vi "Pump Status Pump Module.vi"(8 "error in (no error)":errorcluster, 11 "?":T1={"State"=enum."Idle", "Start Time"=timestamp(0 s since 1904-01-01), "Configuration"={"Cycle Period"=0.0, "Ismatech"={"VISA resource name"="", "Simulated?"=FALSE, "Pump Number"=1.0, "Reverse?"=FALSE}, "Masterflex"={"VISA resource name"="", "Simulated?"=FALSE, "Pump Number"=1.0, "Reverse?"=FALSE}, "Manual Entry"=0.0, "VICI Settings"={"VISA resource name"="", "Simulated?"=FALSE, "Pump Letter"="", "Reverse?"=FALSE}, "Output Device"=enum."VICI", "Tacmina Settings"={"Analog DAQ Task"="", "Digital DAQ Task"=""}, "KNF SIMDOS Settings"={"VISA resource name"="", "Simulated?"=TRUE}, "ASIA Pump C"={"ASIA Pump #"=0, "channel"=0, "Simulated"=FALSE}, "FLOM Settings"={"VISA resource name"="", "Simulated?"=TRUE, "Pump Number"=0.0}, "Pump Calibration File"=path "", "Calibration Slope"=0.0, "Calibration Y Intercept"=0.0, "Pump Cal Enum"=0, "SSI PR Settings"={"VISA resource name"="", "Simulated?"=FALSE}}, "Current Time"=timestamp(0 s since 1904-01-01), "First Iteration"=FALSE, "Data"={"Pump Speed"=0.0, "Pump Pressure"=0.0, "Pump Flow"=0.0}, "Process Name"="", "Pump On?"=enum."Off", "Output Error"=FALSE, "Log Started"=FALSE, "Overpressure Alarming"=FALSE} {"Configuration"."ASIA Pump C"."channel" min=0 max=1 step=1; "Configuration"."Masterflex"."Pump Number" min=1.0 max=20.0 step=1.0; "Configuration"."Ismatech"."Pump Number" min=1.0 max=20.0 step=1.0}) -> (0 "error out":errorcluster, 3 "State out":T1={"State"=enum."Idle", "Start Time"=timestamp(0 s since 1904-01-01), "Configuration"={"Cycle Period"=0.0, "Ismatech"={"VISA resource name"="", "Simulated?"=FALSE, "Pump Number"=1.0, "Reverse?"=FALSE}, "Masterflex"={"VISA resource name"="", "Simulated?"=FALSE, "Pump Number"=1.0, "Reverse?"=FALSE}, "Manual Entry"=0.0, "VICI Settings"={"VISA resource name"="", "Simulated?"=FALSE, "Pump Letter"="", "Reverse?"=FALSE}, "Output Device"=enum."Ismatec ISM 831C", "Tacmina Settings"={"Analog DAQ Task"="", "Digital DAQ Task"=""}, "KNF SIMDOS Settings"={"VISA resource name"="", "Simulated?"=TRUE}, "ASIA Pump C"={"ASIA Pump #"=0, "channel"=0, "Simulated"=FALSE}, "FLOM Settings"={"VISA resource name"="", "Simulated?"=TRUE, "Pump Number"=0.0}, "Pump Calibration File"=path "", "Calibration Slope"=0.0, "Calibration Y Intercept"=0.0, "Pump Cal Enum"=0, "SSI PR Settings"={"VISA resource name"="", "Simulated?"=FALSE}}, "Current Time"=timestamp(0 s since 1904-01-01), "First Iteration"=FALSE, "Data"={"Pump Speed"=0.0, "Pump Pressure"=0.0, "Pump Flow"=0.0}, "Process Name"="", "Pump On?"=enum."Off", "Output Error"=FALSE, "Log Started"=FALSE, "Overpressure Alarming"=FALSE} {"Configuration"."ASIA Pump C"."channel" min=0 max=1 step=1; "Configuration"."Masterflex"."Pump Number" min=1.0 max=20.0 step=1.0; "Configuration"."Ismatech"."Pump Number" min=1.0 max=20.0 step=1.0})   [LabVIEW 2018, in "Pump Module.lvlib"]
uses:
  Pump Module.lvlib
  Measure Instrument/State Cluster.ctl
  Measure Instrument/State Enum.ctl
  Pump Module Settings Cluster.ctl
  Ismatec ISM 831C/Controls/Ismatech Settings Cluster.ctl
  Masterflex 7550-30/Controls/Settings Cluster.ctl
  VICI M50 Party Mode/Settings Cluster.ctl
  Measure Instrument/PID 2 Output Enum.ctl
  Tacmina QI/Tacmina QI DAQ Setting.ctl
  KNF Pump/Settings Cluster plus SIMDOS.ctl
  ASIA Pump/Pump Settings.ctl
  FLOM Pump/Settings Cluster.ctl
  SSI PR Class/SSI PR Settings Cluster.ctl
  Tag VIs/Tag FGV Operation Enum.ctl
  Ismatec ISM 831C/Ismatec ISM 831C.lvlib
  Masterflex 7550-30/Masterflex 7550-30.lvlib
  Shared Variables/Dynamic Shared Variables.lvlib
  Measure Instrument/Pump Module Engine.lvlib
  Tacmina QI/Tacmina QI.lvlib
  KNF Pump/KNF SIMDOS.lvlib
  VICI M50 Party Mode/VICI M6 M50 Party Mode.lvlib
  FLOM Pump/FLOM Pump.lvlib
  ASIA Pump.lvlib
  SSI PR Class/SSI PR Pump.lvlib
panel:
  # "Output Instruments"
  # "Output Instruments"
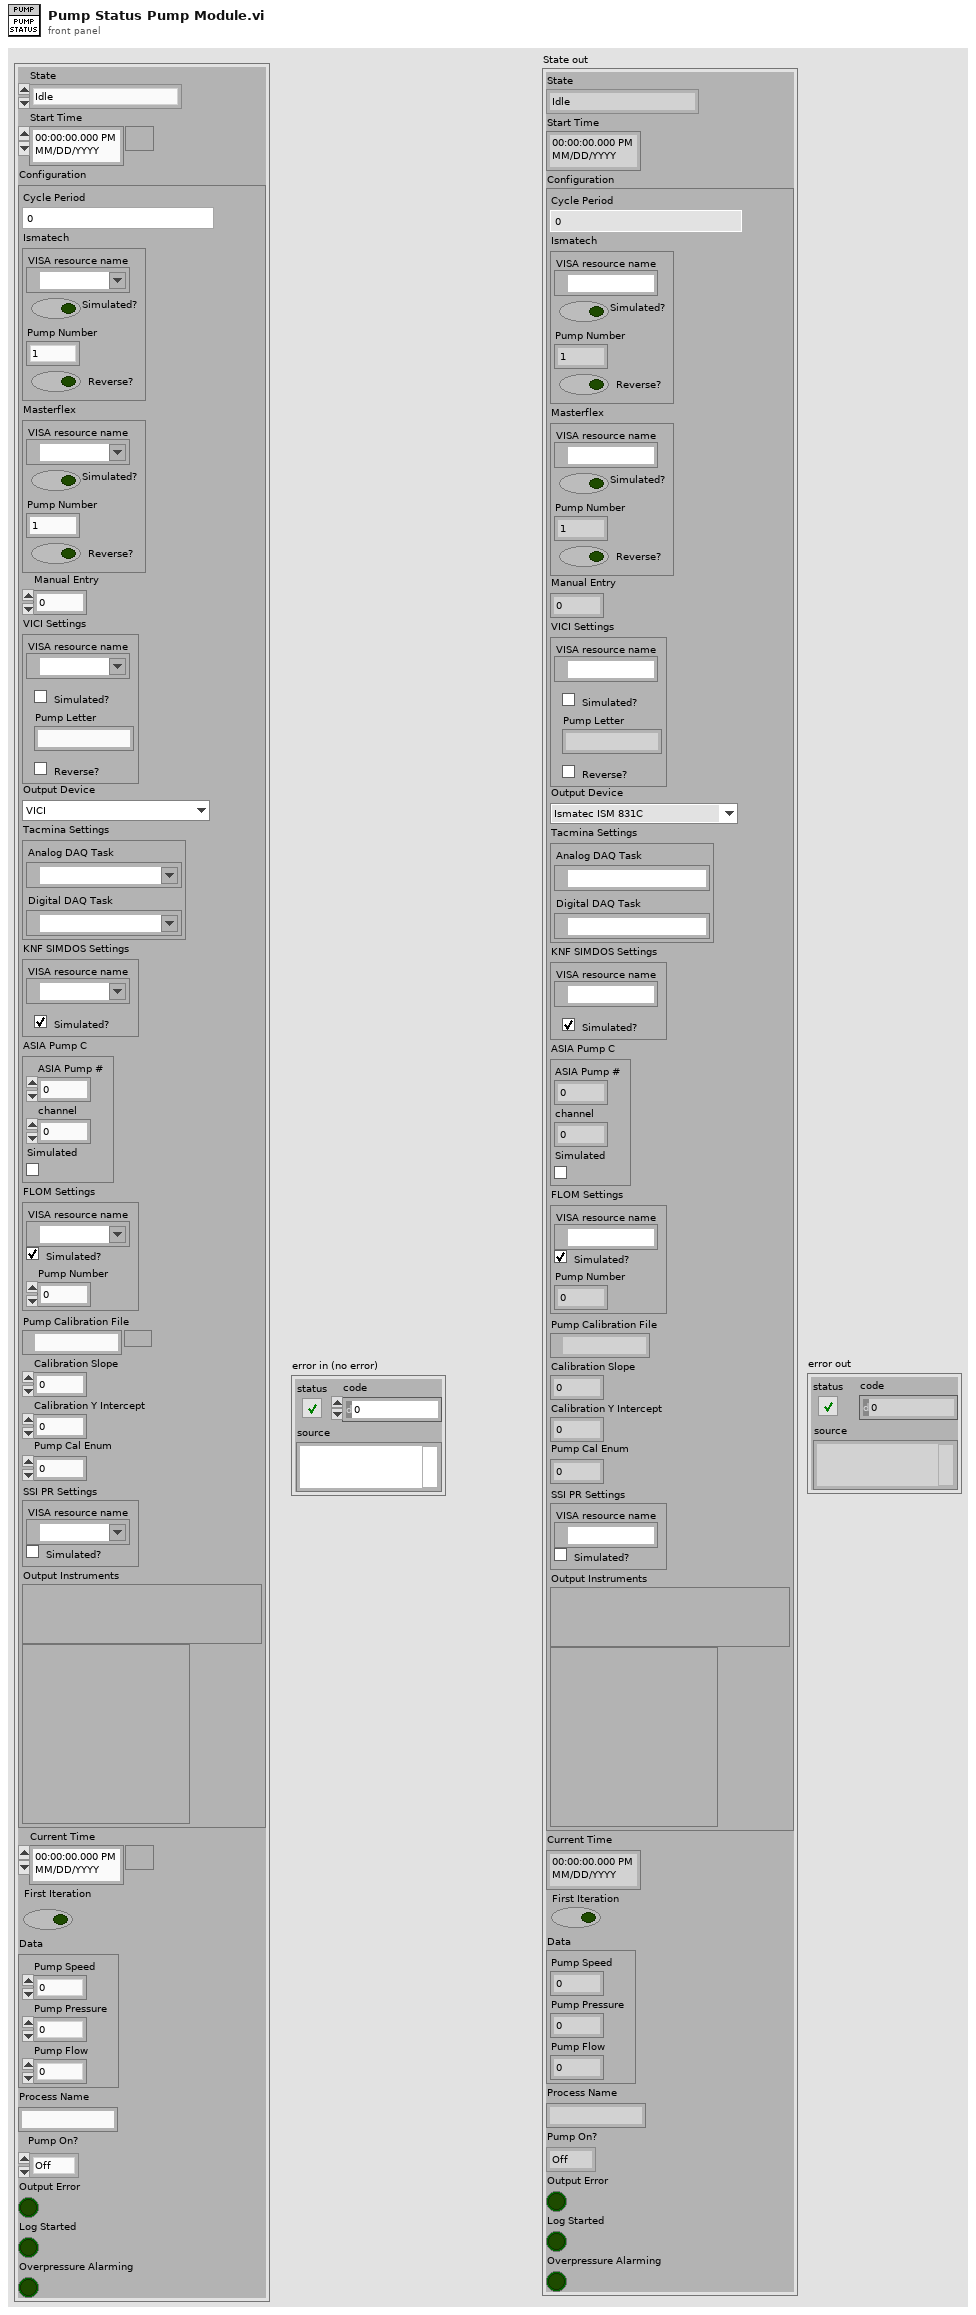
[diagram p1: front panel]
types:
  T1 = typedef "Pump Module.lvlib/Pump Module Engine.lvlib/State Cluster.ctl" = cluster{"State":T2, "Start Time":timestamp, "Configuration":T3, "Current Time":timestamp, "First Iteration":bool, "Data":cluster{"Pump Speed":dbl, "Pump Pressure":dbl, "Pump Flow":dbl}, "Process Name":string, "Pump On?":enum16{"Off", "On", "Not Initialized"}, "Output Error":bool, "Log Started":bool, "Overpressure Alarming":bool}
  T2 = typedef "Pump Module.lvlib/Pump Module Engine.lvlib/State Enum.ctl" = enum16{"Measuring", "Idle", "Paused"}
  T3 = typedef "Pump Module.lvlib/Pump Module Settings Cluster.ctl" = cluster{"Cycle Period":dbl, "Ismatech":T4, "Masterflex":T5, "Manual Entry":dbl, "VICI Settings":T6, "Output Device":T7, "Tacmina Settings":T8, "KNF SIMDOS Settings":T9, "ASIA Pump C":T10, "FLOM Settings":T11, "Pump Calibration File":path, "Calibration Slope":dbl, "Calibration Y Intercept":dbl, "Pump Cal Enum":u16, "SSI PR Settings":T12}
  T4 = typedef "Ismatec ISM 831C.lvlib/Ismatech Settings Cluster.ctl" = cluster{"VISA resource name":refnum<visa-resource-name>, "Simulated?":bool, "Pump Number":dbl, "Reverse?":bool}
  T5 = typedef "Masterflex 7550-30.lvlib/Settings Cluster.ctl" = cluster{"VISA resource name":refnum<visa-resource-name>, "Simulated?":bool, "Pump Number":dbl, "Reverse?":bool}
  T6 = typedef "VICI M6 M50 Party Mode.lvlib/Settings Cluster.ctl" = cluster{"VISA resource name":refnum<visa-resource-name>, "Simulated?":bool, "Pump Letter":string, "Reverse?":bool}
  T7 = typedef "PID 2 Output Enum.ctl" = enum16{"Default", "Ismatec ISM 831C", "Masterflex 7550-30", "VICI", "Tacmina QI", "KNF SIMDOS", "ASIA Type C", "FLOM UI-22-11", "SSI PR"}
  T8 = typedef "Tacmina QI.lvlib/Tacmina QI DAQ Setting.ctl" = cluster{"Analog DAQ Task":refnum<k21>, "Digital DAQ Task":refnum<k21>}
  T9 = typedef "KNF SIMDOS.lvlib/Settings Cluster plus SIMDOS.ctl" = cluster{"VISA resource name":refnum<visa-resource-name>, "Simulated?":bool}
  T10 = typedef "ASIA Pump.lvlib/Pump Settings.ctl" = cluster{"ASIA Pump #":i32, "channel":i32, "Simulated":bool}
  T11 = typedef "FLOM Pump.lvlib/Settings Cluster.ctl" = cluster{"VISA resource name":refnum<visa-resource-name>, "Simulated?":bool, "Pump Number":dbl}
  T12 = typedef "SSI PR Pump.lvlib/SSI PR Settings Cluster.ctl" = cluster{"VISA resource name":refnum<visa-resource-name>, "Simulated?":bool}
  T13 = typedef "Tag FGV Operation Enum.ctl" = enum16{"Init", "Set Notification Queue", "Create Tag", "Commit", "Write Tag (Numeric)", "Write Tag (Boolean)", "Read All Tags", "Read One Tag", "Delete Tag Category", "Set Alarm Parameters (Numeric)", "Set Alarm Parameters (Boolean)", "Enable All Alarms", "Disable All Alarms", "Delete All Tags", "Read Alarms", "Ack Alarm", "Read Alarm Parameters (Numeric)", "Read Alarm Parameters (Boolean)"}
  T14 = typedef "Pump Module.lvlib/Pump Module Tag Names Cluster.ctl" = cluster{"Pump Speed":string, "Pump Flow":string, "Pump Pressure":string, "Output Device Tag":string, "Overpressure Tag":string}
  T15 = cluster{"alarm URL":string, "set time":timestamp, "set user":string, "ack time":timestamp, "ack user":string, "clear time":timestamp, "clear user":string, "setpoint":dbl, "value":dbl, "priority":u32, "alarm area":string, "alarm description":string, "ack comment":string, "event?":bool, "Refnum":u64}[]
  T16 = typedef "Dynamic Shared Variables.lvlib/Alarm Cluster (UI).ctl" = cluster{"Color Box":u32, "Name":string, "Ack":bool}
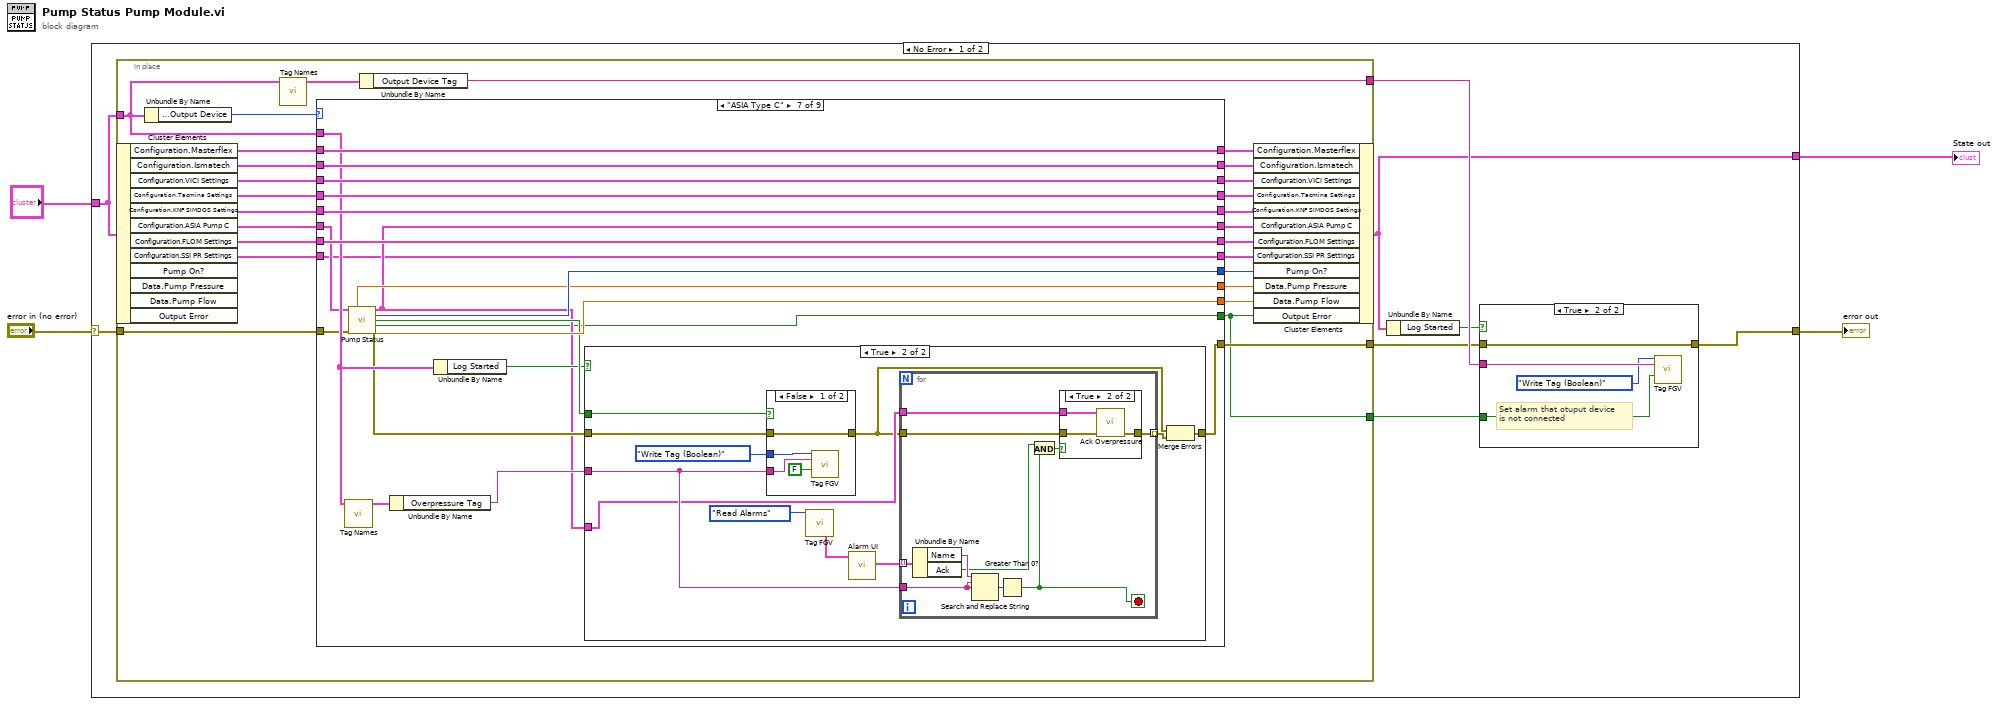
[diagram p0: block diagram]
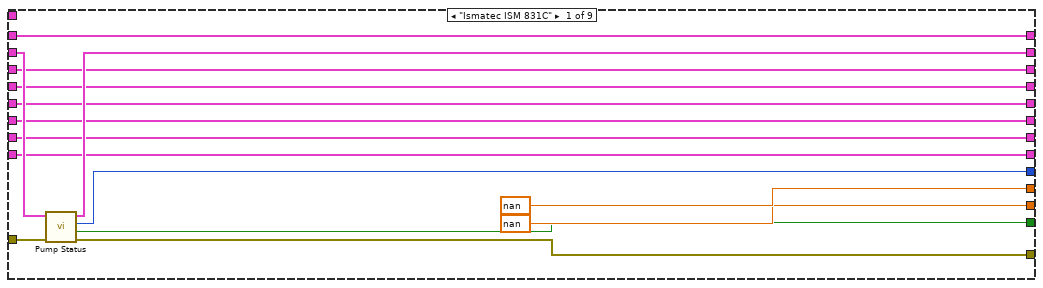
[diagram p2: hidden frame]
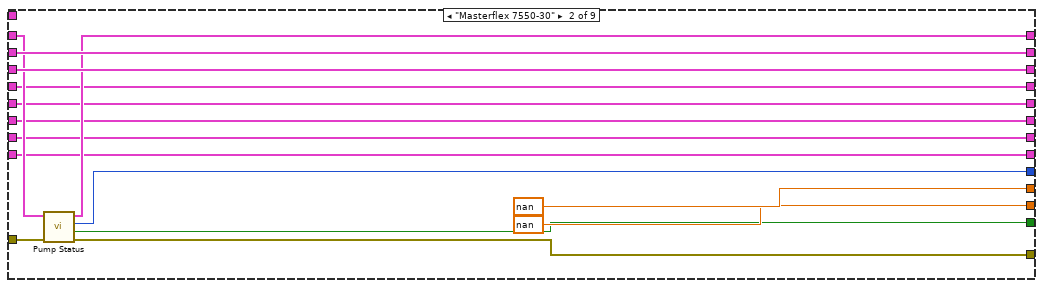
[diagram p3: hidden frame]
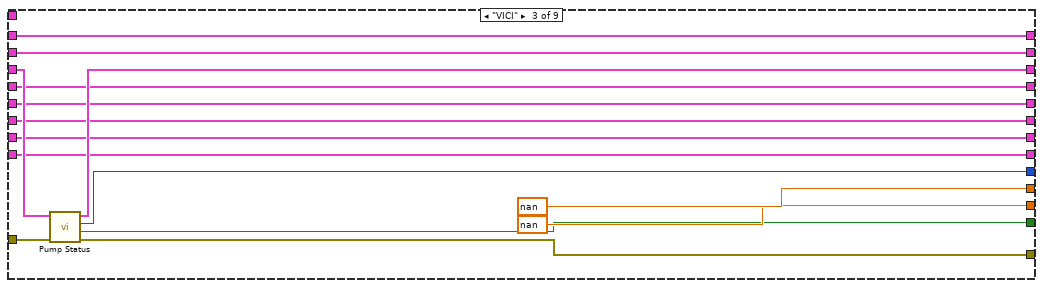
[diagram p4: hidden frame]
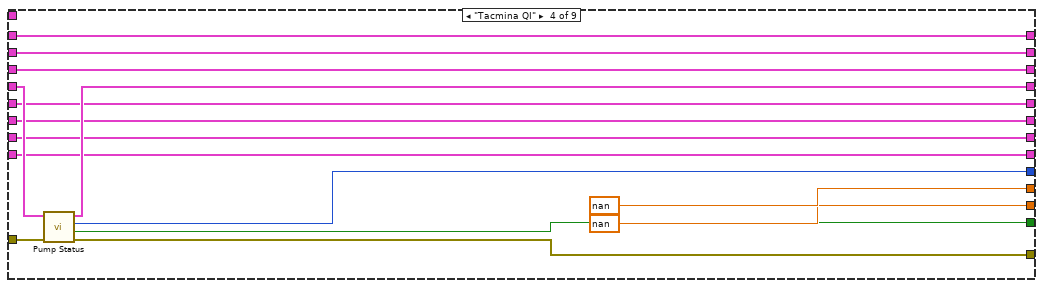
[diagram p5: hidden frame]
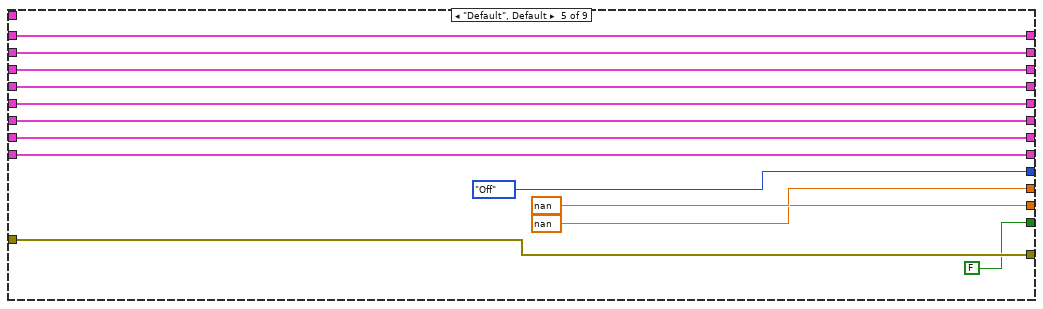
[diagram p6: hidden frame]
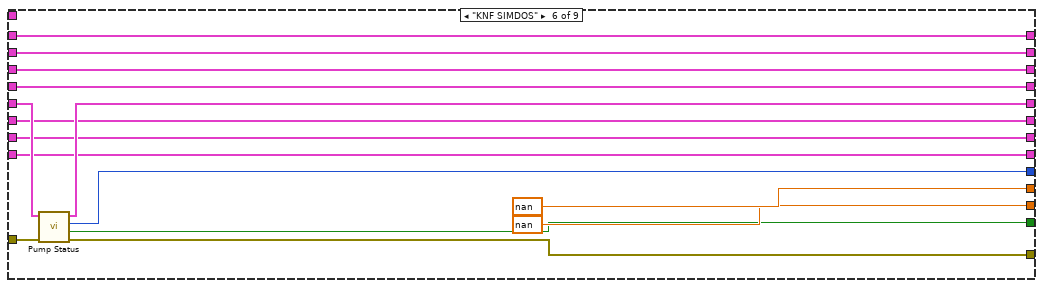
[diagram p7: hidden frame]
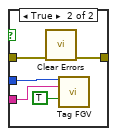
[diagram p10: hidden frame]
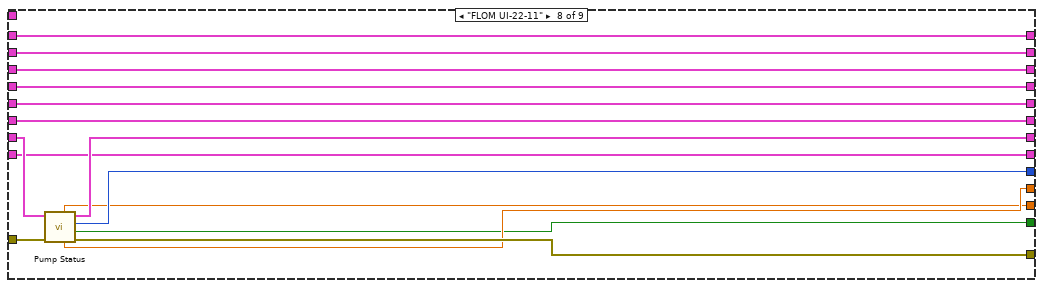
[diagram p11: hidden frame]
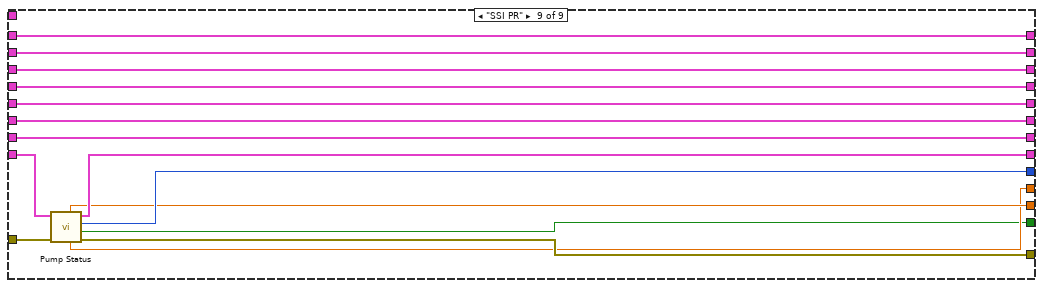
[diagram p12: hidden frame]
diagram:
  n1 = case shown="No Error" "error in (no error)" {
    selector: "error in (no error)" -> [w12 w219]
    tunnel: [w9 w219] -> w3
    tunnel: "?" -> [w6 w218]
    tunnel: [w5 w218] -> w1
    frame No Error {
      n2 = in-place {
        in-place-border: w12 -> [w38]
        in-place-border: [w37] -> w11
        in-place-border: [w36] -> w10
        in-place-border: w6 -> [w33]
        in-place-border: [w24] -> w7
        n3 = in-place-cluster #1(w6) -> ("Configuration.Masterflex"=w32:T5, "Configuration.Ismatech"=w31:T4, "Configuration.VICI Settings"=w30:T6, "Configuration.Tacmina Settings"=w29:T8, "Configuration.KNF SIMDOS Settings"=w28:T9, "Configuration.ASIA Pump C"=w27:T10, "Configuration.FLOM Settings"=w26:T11, "Configuration.SSI PR Settings"=w25:T12)  [unwired: 4 out]
        n4 = Unbundle By Name(w33) -> ("Configuration.Output Device"=w34:T7)
        n5 = call "Tag Names.vi"("State In"=w33) -> ("Pump Module Tag Names"=w35:T14)  [unwired: 8 in, 2 out]
        n6 = case "Selected Device" shown="\"ASIA Type C\"" w34 {
          tunnel: w32 -> [w53 w63 w82 w98 w111 w126 w147 w197 w212]
          tunnel: [w53 w64 w82 w98 w111 w126 w147 w197 w212] -> w23
          tunnel: w31 -> [w50 w68 w83 w97 w110 w125 w146 w196 w211]
          tunnel: [w51 w65 w78 w93 w108 w121 w130 w190 w202] -> w36
          tunnel: w38 -> [w52 w66 w79 w94 w108 w122 w139 w191 w206]
          tunnel: [w49 w68 w83 w97 w110 w125 w146 w196 w211] -> w22
          tunnel: w30 -> [w47 w67 w80 w96 w109 w124 w145 w195 w210]
          tunnel: [w47 w67 w81 w96 w109 w124 w145 w195 w210] -> w21
          tunnel: w29 -> [w48 w62 w77 w95 w107 w123 w144 w194 w209]
          tunnel: [w48 w62 w77 w92 w107 w123 w144 w194 w209] -> w20
          tunnel: [w46 w61 w76 w91 w106 w120 w143 w193 w208] -> w19
          tunnel: w28 -> [w46 w61 w76 w91 w106 w119 w143 w193 w208]
          tunnel: [w45 w59 w75 w90 enum16{"Off", "On", "Not Initialized"}."Off" ("Pump On?") w118 w137 w187 w201] -> w15
          tunnel: [w44 w60 w74 w89 w104 w117 w129 w192 w207] -> w18
          tunnel: w27 -> [w44 w60 w74 w89 w104 w117 w138 w192 w207]
          tunnel: [w43 w58 w73 w88 w103 w116 w142 w189 w205] -> w17
          tunnel: w26 -> [w43 w58 w73 w88 w103 w116 w142 w188 w205]
          tunnel: [nan ("Flow Rate") nan ("Flow Rate") nan ("Flow Rate") nan ("Flow Rate") nan ("Flow Rate") nan ("Flow Rate") w134 w185 w200] -> w13
          tunnel: [nan ("Pressure") nan ("Pressure") nan ("Pressure") nan ("Pressure") nan ("Pressure") nan ("Pressure") w135 w186 w199] -> w14
          tunnel: w33 -> [_ _ _ _ _ _ w140 _ _]
          tunnel: w25 -> [w40 w55 w70 w85 w100 w113 w128 w184 w204]
          tunnel: [w40 w55 w70 w85 w100 w113 w128 w184 w203] -> w16
          tunnel: [w39 w54 w69 w84 FALSE ("Connection Error") w112 w127 w183 w198] -> w24
          frame "Ismatec ISM 831C" {
            n7 = call "Pump Status.vi"("error in (no error)"=w52, "Ismatech Settings"=w50) -> ("error out"=w51:errorcluster, "Connection Error"=w39:bool, "Pump On?"=w45:enum16{"Off", "On", "Not Initialized"}, "Ismatech Settings"=w49:T4)  [unwired: 6 in]
          }
          frame "Masterflex 7550-30" {
            n8 = call "Pump Status.vi"("error in (no error)"=w66, "Masterflex Settings in"=w63) -> ("error out"=w65:errorcluster, "Connection Error"=w54:bool, "Pump On?"=w59:enum16{"Off", "On", "Not Initialized"}, "Masterflex Settings out"=w64:T5)  [unwired: 6 in]
          }
          frame "VICI" {
            n9 = call "Pump Status.vi"("error in (no error)"=w79, "VICI Settings"=w80) -> ("error out"=w78:errorcluster, "Connection Error"=w69:bool, "Pump On?"=w75:enum16{"Off", "On", "Not Initialized"}, "VICI Settings"=w81:T6)  [unwired: 6 in]
          }
          frame "Tacmina QI" {
            n10 = call "Pump Status.vi"("error in"=w94, "Tacmina Settings in"=w95) -> ("error out"=w93:errorcluster, "Connection Error"=w84:bool, "Pump On?"=w90:enum16{"Off", "On", "Not Initialized"}, "Tacmina Settings out"=w92:T8)  [unwired: 6 in]
          }
          frame "Default", Default {
          }
          frame "KNF SIMDOS" {
            n11 = call "Pump Status.vi"("error in (no error)"=w122, "KNF Settings"=w119) -> ("error out"=w121:errorcluster, "Connection Error"=w112:bool, "Pump On?"=w118:enum16{"Off", "On", "Not Initialized"}, "KNF Settings"=w120:T9)  [unwired: 6 in]
          }
          frame "ASIA Type C" {
            n12 = call "Tag Names.vi"("State In"=w140) -> ("Pump Module Tag Names"=w141:T14)  [unwired: 8 in, 2 out]
            n13 = call "Pump Status.vi"("ASIA Pump C Settings in"=w138, "error in (no error)"=w139) -> ("pressure"=w135:dbl, "ASIA Pump C Settings out"=w129:T10, "Pump On?"=w137:enum16{"Off", "On", "Not Initialized"}, "Overpressure"=w133:bool, "Connection Error"=w127:bool, "pumpRate"=w134:dbl, "error out"=w136:errorcluster)  [unwired: 5 in, 2 out]
            n14 = Unbundle By Name(w141) -> ("Overpressure Tag"=w131:string)
            n15 = Unbundle By Name(w140) -> ("Log Started"=w132:bool)
            n16 = case shown="True" w132 {
              tunnel: w131 -> [_ w153]
              tunnel: w136 -> [w148 w159]
              tunnel: w133 -> [_ w158]
              tunnel: [w148 w150] -> w130
              tunnel: w129 -> [_ w152]
              frame False {
              }
              frame True {
                n17 = case shown="False" w158 {
                  tunnel: Tag_FGV_Operation_Enum."Write Tag (Boolean)" ("Operation") -> [w177 w182]
                  tunnel: w153 -> [w176 w181]
                  tunnel: [w175 w179] -> w149
                  tunnel: w159 -> [w175 w180]
                  frame False {
                    n18 = call "Tag FGV.vi"("Operation"=w177, "Tag Name"=w176, "Data"=FALSE) -> ()  [unwired: 5 in, 8 out]
                  }
                  frame True {
                    n19 = call <vilib>:"Clear Errors.vi"("error in (no error)"=w180) -> ("error out"=w179:errorcluster)  [unwired: 5 in, 1 out]
                    n20 = call "Tag FGV.vi"("Operation"=w182, "Tag Name"=w181, "Data"=TRUE) -> ()  [unwired: 5 in, 8 out]
                  }
                }
                n21 = call "Tag FGV.vi"("Operation"=Tag_FGV_Operation_Enum."Read Alarms") -> ("alarms"=w155:T15)  [unwired: 7 in, 7 out]
                n22 = call "Alarm UI.vi"("alarms"=w155) -> ("UI Alarms"=w154:T16[])  [unwired: 9 in, 1 out]
                n23 = for {
                  tunnel: w154 -> [w169] mode=indexing
                  tunnel: w153 -> [w166]
                  tunnel: w152 -> [w165]
                  tunnel: [w164] -> w151 mode=indexing
                  tunnel: w149 -> [w163]
                  stop <- w161 stop-if-true
                  n24 = Unbundle By Name(w169) -> ("Name"=w168:string, "Ack"=w160:bool)
                  n25 = Search and Replace String(input string=w168, search string=w166, replace string=w166) -> (number of replacements=w167:i32)  [unwired: 5 in, 3 out]
                  n26 = Greater Than 0?(x=w167) -> (x > 0?=w161:bool)
                  n27 = And(x=w160, y=w161) -> (x .and. y?=w162:bool)
                  n28 = case shown="True" w162 {
                    tunnel: w165 -> [_ w173]
                    tunnel: [w170 w172] -> w164
                    tunnel: w163 -> [w170 w171]
                    frame False {
                    }
                    frame True {
                      n29 = call "Ack Overpressure.vi"("error in (no error)"=w171, "ASIA Pump C Settings in"=w173) -> ("error out"=w172:errorcluster)  [unwired: 9 in]
                    }
                  }
                }
                n30 = Merge Errors(w149, w151) -> (w150:errorcluster)
              }
            }
          }
          frame "FLOM UI-22-11" {
            n31 = call "Pump Status.vi"("error in (no error)"=w191, "FLOM Settings In"=w188) -> ("error out"=w190:errorcluster, "Connection Error"=w183:bool, "Pump On?"=w187:enum16{"Off", "On", "Not Initialized"}, "FLOM Settings Out"=w189:T11, "Pressure"=w186:dbl, "Flow Rate"=w185:dbl)  [unwired: 4 in]
          }
          frame "SSI PR" {
            n32 = call "Pump Status.vi"("error in (no error)"=w206, "SSI PR Settings"=w204) -> ("error out"=w202:errorcluster, "Connection Error"=w198:bool, "Pump On?"=w201:enum16{"Off", "On", "Not Initialized"}, "SSI PR Settings"=w203:T12, "Pressure"=w199:dbl, "Flow"=w200:dbl)  [unwired: 4 in]
          }
        }
        n33 = Unbundle By Name(w35) -> ("Output Device Tag"=w37:string)
        n34 = in-place-cluster #1("Configuration.Masterflex"=w23, "Configuration.Ismatech"=w22, "Configuration.VICI Settings"=w21, "Configuration.Tacmina Settings"=w20, "Configuration.KNF SIMDOS Settings"=w19, "Configuration.ASIA Pump C"=w18, "Configuration.FLOM Settings"=w17, "Configuration.SSI PR Settings"=w16, "Pump On?"=w15, "Data.Pump Pressure"=w14, "Data.Pump Flow"=w13, "Output Error"=w24) -> (w5:T1)
      }
      n35 = Unbundle By Name(w5) -> ("Log Started"=w8:bool)
      n36 = case shown="True" w8 {
        tunnel: w11 -> [_ w217]
        tunnel: w10 -> [w213 w216]
        tunnel: [w213 w216] -> w9
        tunnel: w7 -> [_ w214]
        frame False {
        }
        frame True {
          # "Set alarm that otuput device\nis not connected"
          n37 = call "Tag FGV.vi"("Operation"=Tag_FGV_Operation_Enum."Write Tag (Boolean)", "Tag Name"=w217, "Data"=w214) -> ()  [unwired: 5 in, 8 out]
        }
      }
    }
    frame Error {
    }
  }
  "error out" <- w3
  "State out" <- w1
